vi "MDPtr Unpack Waveform.vi"(10 "error in (no error)":errorcluster, 11 "HexStrPtr":T1) -> (1 "String Attribute":string, 2 "error out":errorcluster, 3 "waveform":waveform(dbl))   [LabVIEW 2017, in "MDPtr.lvlib"]
uses:
  MDPtr TypeDef/MDPtr.ctl
  MDPtr.lvlib
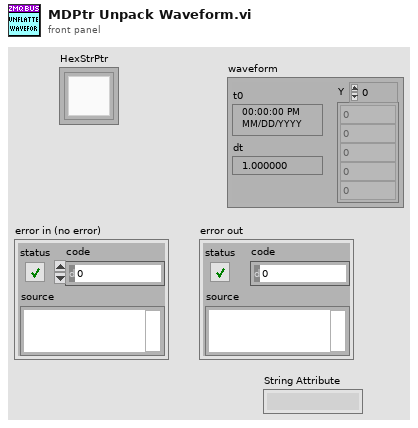
[diagram p1: front panel]
types:
  T1 = typedef "MDPtr.lvlib/MDPtr.ctl" = refnum<k1>
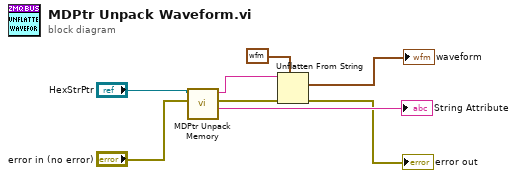
[diagram p0: block diagram]
diagram:
  n1 = call "MDPtr Unpack Memory.vi"("error in (no error)"="error in (no error)", "HexStrPtr"="HexStrPtr") -> ("String Attribute"=→"String Attribute":string, "error out"=w6:errorcluster, "string"=w3:string)  [unwired: 7 in]
  n2 = Unflatten From String(type=waveform(dbl) {"t0"=timestamp(0 s since 1904-01-01), "dt"=1.0, "Y"=[]} ("waveform"), binary string=w3, error in (no error)=w6) -> (value=→"waveform":waveform(dbl), error out=→"error out":errorcluster)  [unwired: 2 in, 1 out]
